vi "Copy to Clipboard.vi"(10 "Text":string) -> ()   [LabVIEW 2009]
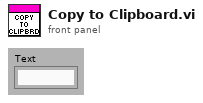
[diagram p1: front panel]
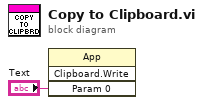
[diagram p0: block diagram]
diagram:
  n1 = invoke class="App" method="Clipboard.Write"("Param 0"="Text") -> ()  [unwired: 3 in, 4 out]
